vi "avg.vi"(1 "Counter":i32, 2 "Flux Avg. Length":u16=25) -> (0 "Boolean":bool)   [LabVIEW 2015]
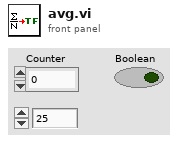
[diagram p1: front panel]
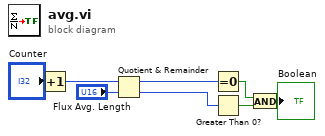
[diagram p0: block diagram]
diagram:
  n1 = Increment(x="Counter") -> (x+1=w7:i32)
  n2 = Quotient & Remainder(x=w7, y="Flux Avg. Length") -> (x-y*floor(x/y)=w3:i32, floor(x/y)=w2:i32)
  n3 = Equal To 0?(x=w3) -> (x = 0?=w4:bool)
  n4 = Greater Than 0?(x=w2) -> (x > 0?=w5:bool)
  n5 = And(x=w4, y=w5) -> (x .and. y?=→"Boolean":bool)
